vi "uTransport_uActor_Create.vi"(8 "error in (no error)":errorcluster) -> (0 "error out":errorcluster, 3 "uTransport_uActor out":refnum<class "uTransport_uActor.lvclass">)   [LabVIEW 2021, in "uFramework.lvlib" / "uTransport_uActor.lvclass"]
uses:
  uTransport_uActor.lvclass
  uMsg/uMsg.lvclass
  uTransport_uActor.lvclass/uTransport_uActor.ctl
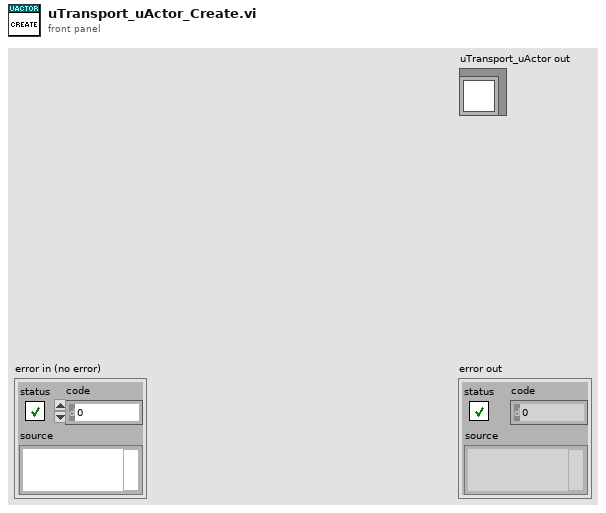
[diagram p1: front panel]
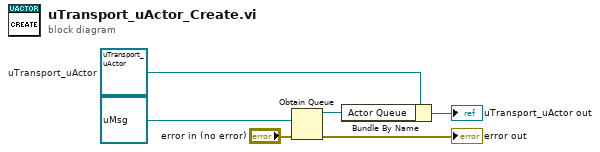
[diagram p0: block diagram]
diagram:
  w4 = refnum<class "uTransport_uActor.lvclass"> refnum  # uTransport_uActor
  n1 = Obtain Queue(element data type=refnum<class "uMsg.lvclass"> refnum ("uTransport.lvlib:uMsg.lvclass"), error in (no error)="error in (no error)") -> (queue out=w3:refnum<queue>, error out=→"error out":errorcluster)  [unwired: 3 in, 1 out]
  n2 = Bundle By Name(cluster=w4, "Actor Queue"=w3) -> (→"uTransport_uActor out":refnum<class "uTransport_uActor.lvclass">)
